vi "asdk Reset.vi"(8 "error in (no error)":errorcluster, 11 "pDm":u64) -> (0 "error out":errorcluster, 3 "pDm out":u32)   [LabVIEW 2017, in "ASDK.lvlib"]
doc: "ASDK_API COMPL_STAT asdkReset( asdkDM *pDm );"
uses:
  ASDK.lvlib
  ASDK.dll
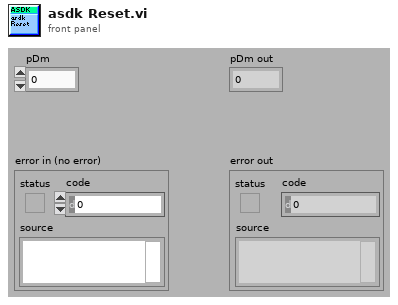
[diagram p1: front panel]
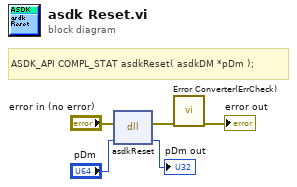
[diagram p0: block diagram]
diagram:
  # "ASDK_API COMPL_STAT asdkReset( asdkDM *pDm );"
  n1 = dll-call lib="ASDK.*" fn="asdkReset"(error in="error in (no error)", "pDm"="pDm") -> (error out=w2:errorcluster, "pDm"=→"pDm out":u32)  [unwired: 3 in, 1 out]
  n2 = call "Error Converter(ErrCheck).vi"("error in (no error)"=w2) -> ("error out"=→"error out":errorcluster)  [unwired: 10 in]
